vi "DriveForDistanceMotionProfile.vi"(11 "Distance":dbl) -> ()   [LabVIEW 2016]
panel:
  in  "error in":errorcluster
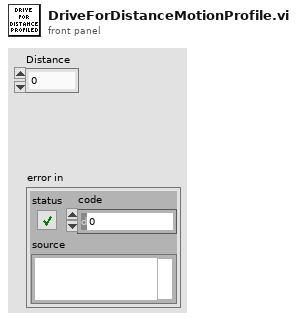
[diagram p1: front panel]
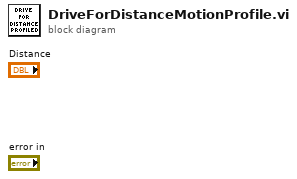
[diagram p0: block diagram]
diagram:
